vi "Set all 0s to previous value (1).vi"(11 "Original Array":dbl[](array[numeric])) -> (3 "Modified Array":dbl[](array[numeric]))   [LabVIEW 2016]
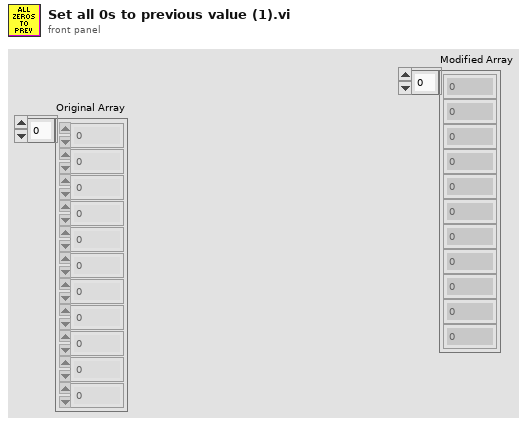
[diagram p1: front panel]
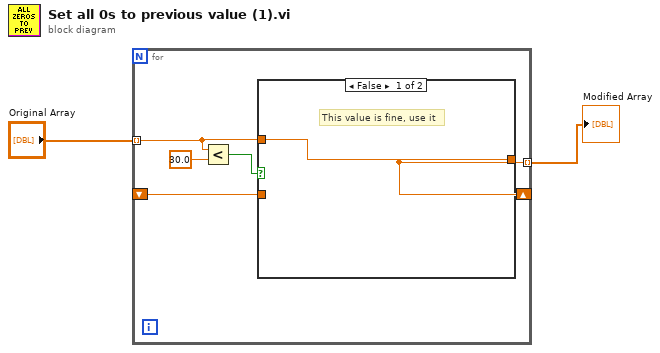
[diagram p0: block diagram]
diagram:
  n1 = for {
    tunnel: "Original Array" -> [w5] mode=indexing
    shift-right: [w3] -> _
    shift-left: _ -> [w4]
    tunnel: [w3] -> w1 mode=indexing
    n2 = Less?(x=w5, y=30.0) -> (x < y?=w6:bool)
    n3 = case shown="False" w6 {
      tunnel: [w8 w9] -> w3
      tunnel: w5 -> [w8 _]
      tunnel: w4 -> [_ w9]
      frame False {
        # "This value is fine, use it"
      }
      frame True {
        # "This is a value close to 0\nSet it to be the same as the value before"
      }
    }
  }
  "Modified Array" <- w1
